vi "Acel_calib_frequency.vi"(5 "Pattern frequency (Hz)":dbl, 6 "Frecuencia\nmuestreo":dbl, 7 "Acel Cal measurements in":sgl[][](array[numeric])) -> (0 "Measurements OK":bool[](array[boolean]), 1 "Valid frequency":bool, 2 "Reporting2":string, 3 "Acel Cal measurements out":sgl[][](array[numeric]))   [LabVIEW 2015]
uses:
  <vilib>/measure/maspectr.llb/FFT Spectrum (Mag-Phase) for 1 Chan.vi
  <vilib>/measure/NI_MAPro.lvlib
  <vilib>/Analysis/NI_AALBase.lvlib
panel:
  out "Mean\nfrequency":dbl format="%0.2f"
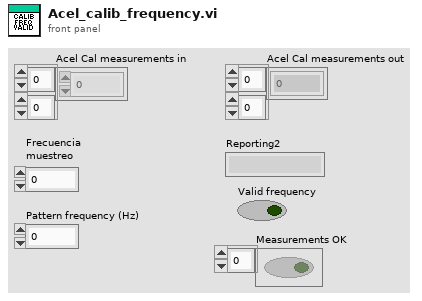
[diagram p1: front panel]
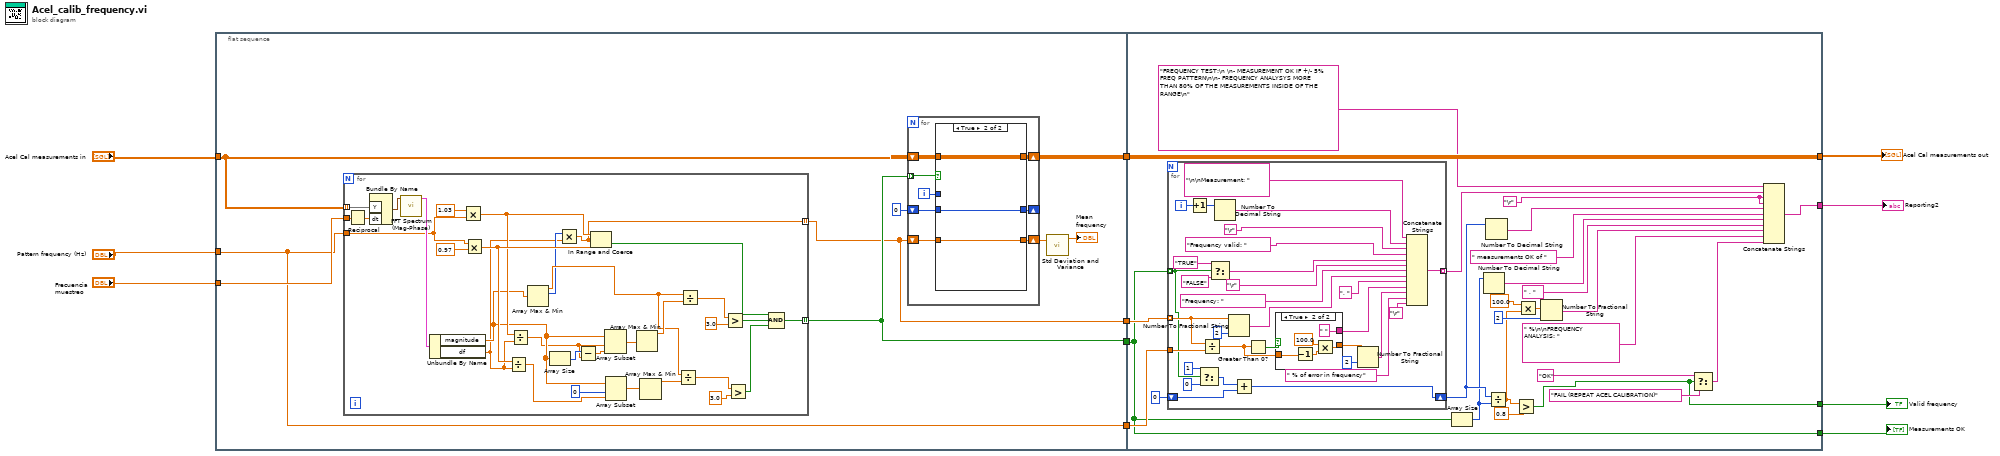
[diagram p0: block diagram]
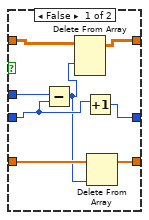
[diagram p2: hidden frame]
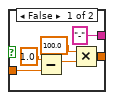
[diagram p3: hidden frame]
diagram:
  n1 = flat-sequence {
    tunnel: "Acel Cal measurements in" -> [w18]
    tunnel: "Frecuencia\nmuestreo" -> [w15]
    tunnel: "Pattern frequency (Hz)" -> [w12]
    tunnel: [w20] -> w11
    tunnel: [w14] -> w10
    tunnel: [w13] -> w9
    tunnel: [w12] -> w8
    tunnel: w11 -> [w97]
    tunnel: w10 -> [w79]
    tunnel: w9 -> [w96]
    tunnel: w8 -> [w95]
    tunnel: [w97] -> w2
    tunnel: [w81] -> w5
    tunnel: [w80] -> w6
    tunnel: [w79] -> w7
    frame #0 {
      n2 = for {
        tunnel: w18 -> [w70] mode=indexing
        tunnel: w15 -> [w69]
        tunnel: w12 -> [w65]
        tunnel: [w46] -> w14 mode=indexing
        tunnel: [w40] -> w13 mode=indexing
        n3 = Reciprocal(x=w69) -> (1/x=w71:dbl)
        n4 = Bundle By Name("Y"=w70, "dt"=w71) -> (w68:waveform(sgl))  [unwired: 1 in]
        n5 = call-poly <vilib>:"FFT Spectrum (Mag-Phase).vi"("time signal"=w68) -> ("magnitude"=w67:cluster{"f0":dbl, "df":dbl, "magnitude":dbl[]})  [unwired: 6 in, 4 out]
        n6 = Unbundle By Name(w67) -> ("magnitude"=w59:dbl[], "df"=w41:dbl)
        n7 = Multiply(x=1.03, y=w65) -> (x*y=w62:dbl)
        n8 = Multiply(x=w65, y=0.97 ("x")) -> (x*y=w63:dbl)
        n9 = Divide(x=w63, y=w41) -> (x/y=w60:dbl)
        n10 = Divide(x=w62, y=w41) -> (x/y=w57:dbl)
        n11 = Array Max & Min(array=w59) -> (max value=w52:dbl, max index (indices)=w42:i32)  [unwired: 2 out]
        n12 = Array Size(array=w59) -> (size(s)=w58:i32)
        n13 = Multiply(x=w42, y=w41) -> (x*y=w40:dbl)
        n14 = Subtract(x=w58, y=w57) -> (x-y=w56:dbl)
        n15 = In Range and Coerce(upper limit=w62, x=w40, lower limit=w63) -> (In Range?=w45:bool)  [unwired: 1 out]
        n16 = Array Subset(array=w59, index=w57, length=w56) -> (w55:dbl[])
        n17 = Array Subset(array=w59, index=0, length=w60) -> (w54:dbl[])
        n18 = Array Max & Min(array=w55) -> (max value=w53:dbl)  [unwired: 3 out]
        n19 = Array Max & Min(array=w54) -> (max value=w51:dbl)  [unwired: 3 out]
        n20 = Divide(x=w52, y=w51) -> (x/y=w49:dbl)
        n21 = Divide(x=w52, y=w53) -> (x/y=w50:dbl)
        n22 = Greater?(x=w50, y=3.0) -> (0:w44:bool)
        n23 = Greater?(x=w49, y=3.0) -> (0:w43:bool)
        n24 = Compound Arithmetic op=AND(w45, w44, w43) -> (w46:bool)
      }
      n25 = for {
        shift-right: [w27] -> w20
        shift-left: w18 -> [w28]
        tunnel: w14 -> [w26] mode=indexing
        shift-right: [w23] -> _
        shift-left: 0 ("index of element") -> [w24]
        shift-right: [w21] -> w17
        shift-left: w13 -> [w22]
        i -> [w25]
        n26 = case shown="True" w26 {
          tunnel: w28 -> [w36 w39]
          tunnel: [w35 w39] -> w27
          tunnel: w25 -> [w34 _]
          tunnel: w24 -> [w33 w38]
          tunnel: [w32 w38] -> w23
          tunnel: w22 -> [w31 w37]
          tunnel: [w29 w37] -> w21
          frame False {
            n27 = Subtract(x=w34, y=w33) -> (x-y=w30:i32)
            n28 = Delete From Array(array=w36, index (row)=w30) -> (array with subset deleted=w35:sgl[][])  [unwired: 2 in, 1 out]
            n29 = Increment(x=w33) -> (x+1=w32:i32)
            n30 = Delete From Array(array=w31, index=w30) -> (array with subset deleted=w29:dbl[])  [unwired: 1 in, 1 out]
          }
          frame True {
          }
        }
      }
      n31 = call <vilib>:"Std Deviation and Variance.vi"("X"=w17) -> ("mean"=→"Mean\nfrequency":dbl)  [unwired: 1 in, 2 out]
    }
    frame #1 {
      w76 = "\r"
      n32 = for {
        tunnel: w79 -> [w105] mode=indexing
        tunnel: w96 -> [w124] mode=indexing
        tunnel: w95 -> [w123]
        tunnel: [w106] -> w93 mode=indexing
        shift-right: [w100] -> w91
        shift-left: 0 -> [w101]
        i -> [w126]
        n33 = Increment(x=w126) -> (x+1=w125:i32)
        n34 = Select(t=1, s=w105, f=0) -> (s? t:f=w102:i32)
        n35 = Divide(x=w124, y=w123) -> (x/y=w121:dbl)
        n36 = Select(t="TRUE", s=w105, f="FALSE") -> (s? t:f=w115:string)
        n37 = Number To Decimal String(number=w125) -> (decimal integer string=w118:string)  [unwired: 1 in]
        n38 = Number To Fractional String(number=w124, precision (6)=i16 2) -> (F-format string=w112:string)  [unwired: 2 in]
        n39 = Add(x=w102, y=w101) -> (x+y=w100:i32)
        n40 = Greater Than 0?(x=w121) -> (x > 0?=w122:bool)
        n41 = case shown="True" w122 {
          tunnel: w121 -> [w134 w136]
          tunnel: [w130 w138] -> w120
          tunnel: ["-" " "] -> w110
          frame False {
            n42 = Subtract(x=1.0, y=w134) -> (x-y=w132:dbl)
            n43 = Multiply(x=100.0, y=w132) -> (x*y=w130:dbl)
          }
          frame True {
            n44 = Decrement(x=w136) -> (x-1=w137:dbl)
            n45 = Multiply(x=100.0, y=w137) -> (x*y=w138:dbl)
          }
        }
        n46 = Number To Fractional String(number=w120, precision (6)=i16 2) -> (F-format string=w109:string)  [unwired: 2 in]
        n47 = Concatenate Strings("\n\nMeasurement: ", w118, "\r", "Frequency valid: ", w115, "\r", "Frequency: ", w112, ", ", w110, w109, " % of error in frequency", "\r") -> (w106:string)
      }
      n48 = Array Size(array=w79) -> (size(s)=w90:i32)
      n49 = Number To Decimal String(number=w90) -> (decimal integer string=w85:string)  [unwired: 1 in]
      n50 = Number To Decimal String(number=w91) -> (decimal integer string=w77:string)  [unwired: 1 in]
      n51 = Divide(x=w91, y=w90) -> (x/y=w74:dbl)
      n52 = Greater?(x=w74, y=0.8) -> (0:w80:bool)
      n53 = Multiply(x=100.0, y=w74) -> (x*y=w73:dbl)
      n54 = Number To Fractional String(number=w73, precision (6)=i16 2) -> (F-format string=w84:string)  [unwired: 2 in]
      n55 = Select(t="OK", s=w80, f="FAIL (REPEAT ACEL CALIBRATION)") -> (s? t:f=w82:string)
      n56 = Concatenate Strings("FREQUENCY TEST:\n \n- MEASUREMENT OK IF +/- 5% FREQ PATTERN\n\n- FREQUENCY ANALYSYS MORE THAN 80% OF THE MEASUREMENTS INSIDE OF THE RANGE\n", w93, w76, w76, w77, " measurements OK of ", w85, " , ", w84, " %\n\nFREQUENCY ANALYSIS: ", w82) -> (w81:string)
    }
  }
  "Measurements OK" <- w7
  "Valid frequency" <- w6
  "Reporting2" <- w5
  "Acel Cal measurements out" <- w2
